vi "LJM_eWriteAddressArray.vi"(0 "Handle In":i32, 5 "Address":i32, 7 "Type":i32, 9 "aValues":dbl[](array[numeric]) format="%.2f", 11 "error in":errorcluster, 13 "NumValues":i32) -> (4 "Handle Out":i32, 14 "ErrorAddress":i32, 15 "error out":errorcluster)   [LabVIEW 2024]
uses:
  labjackm.dll
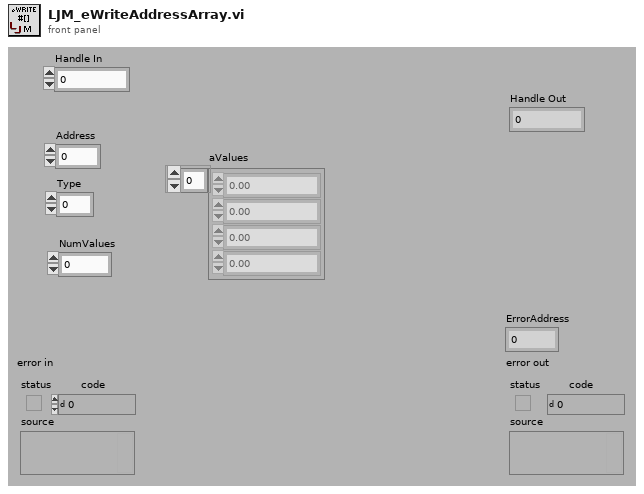
[diagram p1: front panel]
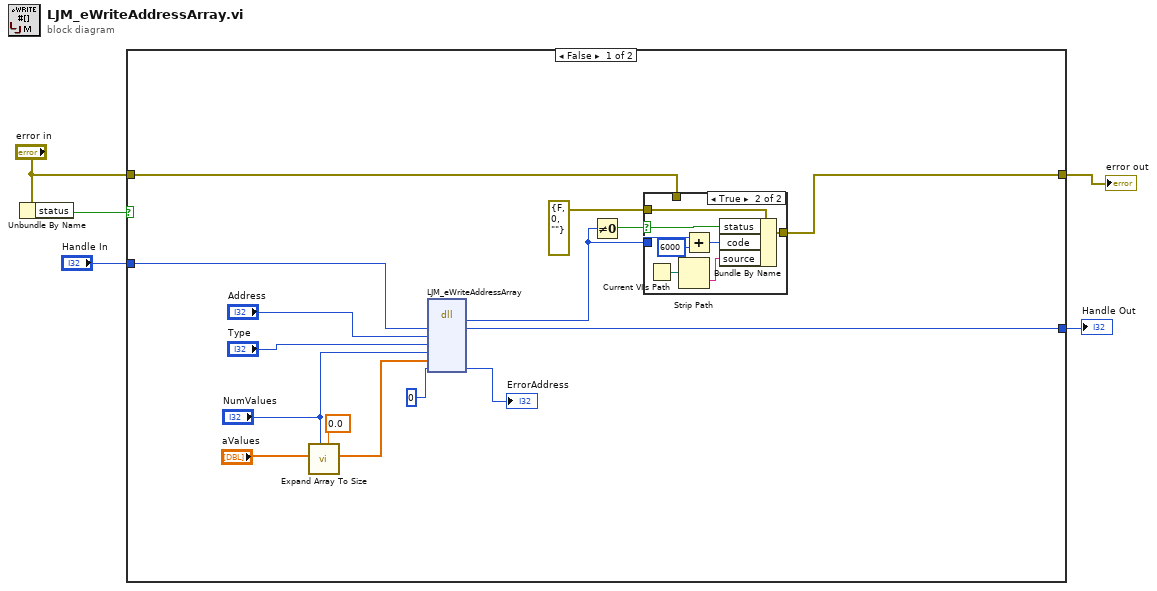
[diagram p0: block diagram]
diagram:
  n1 = Unbundle By Name("error in") -> ("status"=w5:bool)
  n2 = case shown="False" w5 {
    tunnel: "error in" -> [w17 w31]
    tunnel: [w16 w31] -> w3
    tunnel: "Handle In" -> [w11 w30]
    tunnel: [w10 w30] -> w1
    frame False {
      n3 = call "Expand Array To Size.vi"("Default Value"=0.0, "# Elements"="NumValues", "DBL Array In"="aValues") -> ("DBL Array Out"=w15:dbl[])  [unwired: 4 in, 4 out]
      n4 = dll-call lib="labjackm.dll" fn="LJM_eWriteAddressArray"("Handle"=w11, "Address"="Address", "Type"="Type", "NumValues"="NumValues", "aValues"=w15, "ErrorAddress"=u32 0 ("ErrorFrame")) -> (w20:i32, "Handle"=w10:i32, "ErrorAddress"=→"ErrorAddress":i32)  [unwired: 7 in, 2 out]
      n5 = Not Equal To 0?(x=w20) -> (x != 0?=w19:bool)
      n6 = case shown="True" w19 {
        selector: w19 -> [_ w28]
        tunnel: [w21 w29] -> w16
        tunnel: errorcluster {"status"=FALSE, "code"=0, "source"=""} ("error IO") -> [_ w27]
        tunnel: w20 -> [_ w23]
        tunnel: w17 -> [w21 _]
        frame False {
        }
        frame True {
          n7 = Current VI's Path() -> (path=w25:path)
          n8 = Strip Path(path=w25) -> (name=w26:string)  [unwired: 1 out]
          n9 = Add(x=w23, y=6000) -> (x+y=w24:i32)
          n10 = Bundle By Name(cluster=w27, "status"=w28, "code"=w24, "source"=w26) -> (w29:errorcluster)
        }
      }
    }
    frame True {
    }
  }
  "error out" <- w3
  "Handle Out" <- w1
